vi "Finalize.vi"(8 "error in (no error)":errorcluster, 11 "Log Producer":refnum<class "Log Producer.lvclass">) -> (0 "error out":errorcluster, 2 "Logger":refnum<class "Logger Interface.lvclass">, 3 "Default Producer":refnum<class "Log Producer.lvclass">)   [LabVIEW 2020, in "Ballard ARINC 429 Engine.lvlib" / "Implementation.lvlib" / "Word Logging.lvlib" / "Log Producer.lvclass"]
uses:
  Log Producer.lvclass
  Logger Interface/Logger Interface.lvclass
  Log Producer.lvclass/Log Producer.ctl
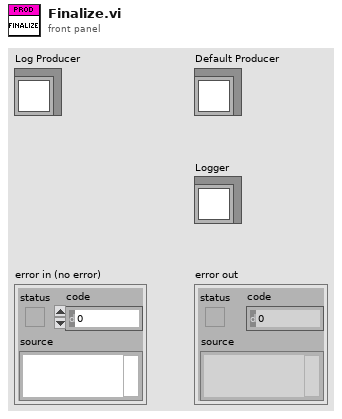
[diagram p1: front panel]
types:
  T1 = typedef "Ballard ARINC 429 Engine.lvlib/Implementation.lvlib/Word Logging.lvlib/Logger Data Reference.ctl" = refnum<data-value>
  T2 = cluster{"Logger Interface":refnum<class "Logger Interface.lvclass">}
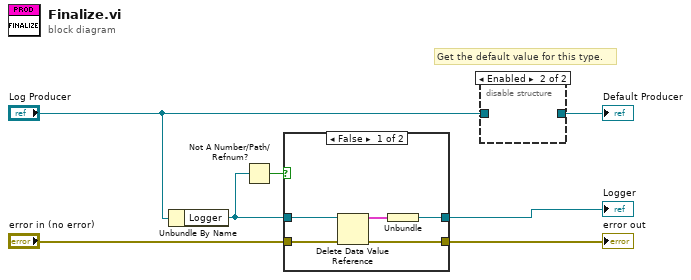
[diagram p0: block diagram]
diagram:
  # "Get the default value for this type."
  n1 = Unbundle By Name("Log Producer") -> ("Logger"=w2:T1)
  n2 = Not A Number/Path/Refnum?(number/path/refnum=w2) -> (NaN/Path/Refnum?=w3:bool)
  n3 = case shown="False" w3 {
    tunnel: [w10 w13] -> w5
    tunnel: "error in (no error)" -> [w12 w13]
    tunnel: w2 -> [w11 _]
    tunnel: [w8 _] -> w1
    frame False {
      n4 = Delete Data Value Reference(data value reference=w11, error in=w12) -> (data value=w9:T2, error out=w10:errorcluster)
      n5 = Unbundle(w9) -> ("Logger Interface"=w8:refnum<class "Logger Interface.lvclass">)
    }
    frame True {
    }
  }
  "error out" <- w5
  "Logger" <- w1
  n6 = disable-structure shown="Enabled" {
    disable-tunnel: "Log Producer" -> [w14 _]
    disable-tunnel: [w14 _] -> w7
    frame Disabled {
    }
    frame Enabled {
    }
  }
  "Default Producer" <- w7
